vi "TransformToJacob.vi"(1 "Transform":T1) -> (0 "Jacobian":T1)   [LabVIEW 2017, in "NI_Kinematics.lvlib"]
uses:
  <vilib>/robotics/Kinematics/NI_Kinematics.lvlib
  <vilib>/Analysis/Matrix/Datatypes/RealMatrix.ctl
  <vilib>/Analysis/NI_AALPro.lvlib
  <vilib>/Analysis/Matrix/NI_Matrix.lvlib
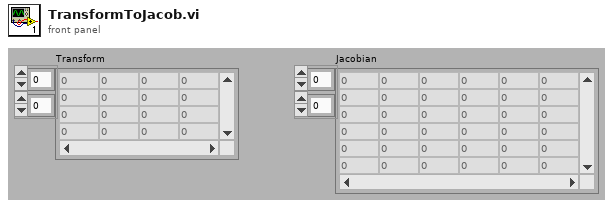
[diagram p1: front panel]
types:
  T1 = typedef "NI_Matrix.lvlib/RealMatrix.ctl" = dbl[][]
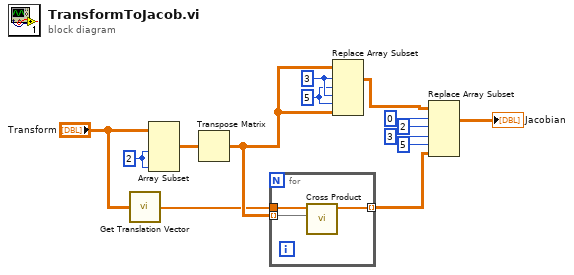
[diagram p0: block diagram]
diagram:
  w12 = 5 ("row N")
  w13 = 3 ("number of rows")
  w14 = 2 ("row N")
  n1 = call <vilib>:"Get Translation Vector.vi"("transform"="Transform") -> ("translation vector"=w1:dbl[])
  n2 = Array Subset(array="Transform", length (row)=w14, length (col)=w14) -> (w4:T1)  [unwired: 2 in]
  n3 = Transpose Matrix(1:w4) -> (0:w3:T1)
  n4 = for {
    tunnel: [w15] -> w5 mode=indexing
    tunnel: w3 -> [w16] mode=indexing
    tunnel: w1 -> [w17]
    n5 = call <vilib>:"Cross Product.vi"("B Vector"=w16, "A Vector"=w17) -> ("Cross Product"=w15:dbl[])  [unwired: 8 in, 1 out]
  }
  n6 = Replace Array Subset(array=w3, new element=w3, index (dim 0)=w13, index (dim 1)=w12, index (dim 2)=w13, index (dim 3)=w12) -> (w11:T1)
  n7 = Replace Array Subset(array=w11, new element=w5, index (dim 0)=0 ("number of rows"), index (dim 1)=2 ("number of rows"), index (dim 2)=3 ("number of rows"), index (dim 3)=5 ("row N")) -> (→"Jacobian":T1)
